vi "N9030B_8257D_0916.vi"() -> ()   [LabVIEW 2017]
uses:
  <vilib>/picture/cartesn2.llb/XY Plot Type.ctl
  <vilib>/Utility/file.llb/Write Delimited Spreadsheet (DBL).vi
  <vilib>/Utility/file.llb/Write Delimited Spreadsheet (string).vi
  <instrlib>/Keysight XSAn/Keysight XSAn.lvlib
panel:
  in  "XY Plot Cosmetics":T2(array[cluster])=[{"Color Box"=3381759, "plot type"=enum."connected squares", "baseline"=0.0}, {"Color Box"=6618880, "plot type"=enum."connected points", "baseline"=0.0}, {"Color Box"=16768018, "plot type"=enum."connected circles", "baseline"=0.0}]
  out "?":picture
  in  "csv header":string[](array[string])
  in  "folder name":string
  out "element":dbl
  out "sweep":bool
  in  "stop":bool
  in  "Path":path=path "d:/"
  out "actual points":i32
  in  "Array":cluster{"Numeric":dbl, "Numeric 2":dbl}[](array[cluster])
  in  "frequency points":T3 {"point 2 (Hz)" format="%#_6p"; "point 1 (Hz)" format="%#_6p"; "frequency 1 (Hz)" format="%#_6p"}
  in  "Keysight N9030B":refnum<visa-resource-name> caption="resource name"
  in  "8257D":refnum<visa-resource-name>
  in  "8257D":T4={"start frequency (MHz)"=150.0, "frequency spacing (MHz)"=1.0, "stop frequency (MHz)"=250.0, "sweep frequency"=FALSE, "Power level"=0.0}
  out "error out":errorcluster {"code" format="%.0x"}
  in  "Keysight N9030B":T5={"center frequency"=15000.0, "span"=5000.0, "noise floor (dBm)"=0.0} {"span" format="%#_6p"; "center frequency" format="%#_6p"}
  out "amplitude":dbl[](array[numeric])
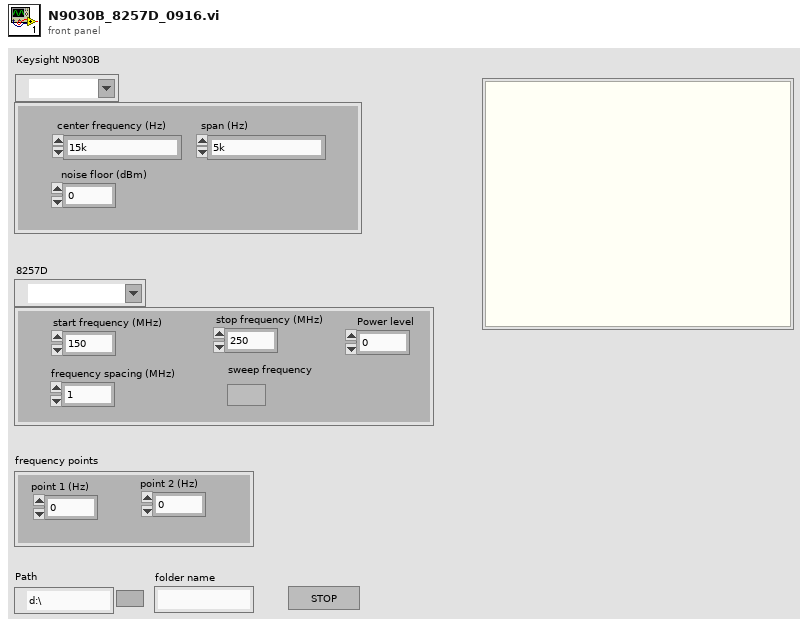
[diagram p1: front panel]
types:
  T1 = typedef "XY Plot Type.ctl" = enum16{"points", "squares", "circles", "connected points", "connected squares", "connected circles", "comb plot", "sized scatter plot", "sized-colored scatter plot", "min-max lines"}
  T2 = cluster{"Color Box":u32, "plot type":T1, "baseline":dbl}[]
  T3 = cluster{"frequency 1 (Hz)":dbl, "point 1 (Hz)":dbl, "point 2 (Hz)":dbl}
  T4 = cluster{"start frequency (MHz)":dbl, "frequency spacing (MHz)":dbl, "stop frequency (MHz)":dbl, "sweep frequency":bool, "Power level":dbl}
  T5 = cluster{"center frequency":dbl, "span":dbl, "noise floor (dBm)":dbl}
  T6 = cluster{"Array":cluster{"Numeric":dbl, "Numeric 2":dbl}[]}
  T7 = cluster{"Array":cluster{"Numeric":dbl, "Numeric 2":dbl}[]}[]
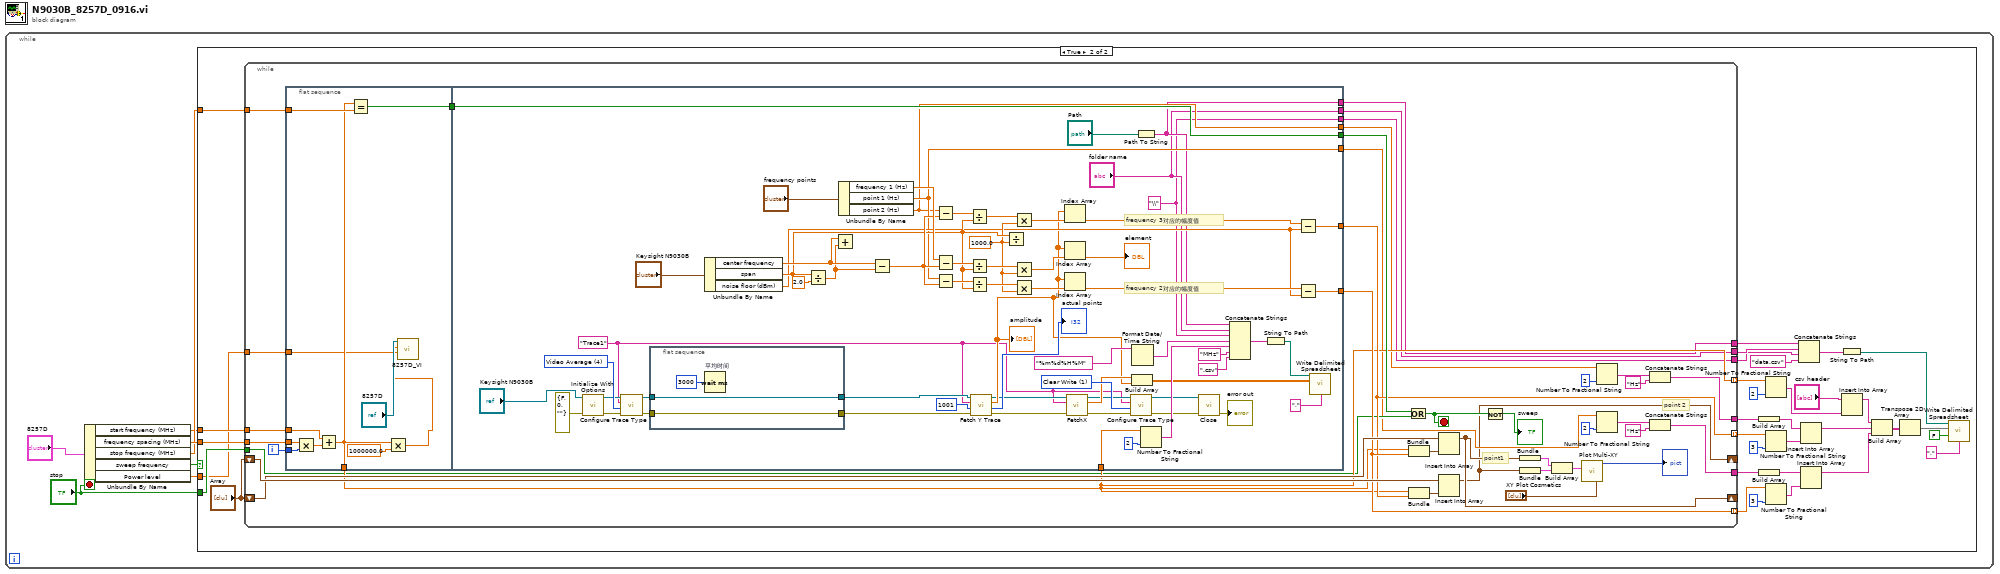
[diagram p0: block diagram]
diagram:
  n1 = while {
    stop <- "stop" stop-if-true
    n2 = Unbundle By Name("8257D") -> ("start frequency (MHz)"=w3:dbl, "frequency spacing (MHz)"=w5:dbl, "stop frequency (MHz)"=w4:dbl, "sweep frequency"=w6:bool, "Power level"=w1:dbl)
    n3 = case shown="True" w6 {
      tunnel: w3 -> [_ w38]
      tunnel: w5 -> [_ w40]
      tunnel: w4 -> [_ w37]
      tunnel: "stop" -> [_ w35]
      tunnel: w1 -> [_ w8]
      frame False {
      }
      frame True {
        n4 = while {
          tunnel: w38 -> [w77]
          tunnel: w40 -> [w76]
          tunnel: w37 -> [w74]
          shift-right: [w50] -> _
          shift-left: "Array" -> [w72]
          shift-right: [w51] -> _
          shift-left: "Array" -> [w71]
          tunnel: [w65] -> w29 mode=indexing
          tunnel: [w64] -> w18 mode=indexing
          tunnel: [w63] -> w24 mode=indexing
          tunnel: w35 -> [w62]
          tunnel: [w57] -> w31
          tunnel: [w52] -> w20
          tunnel: [w44] -> w14
          tunnel: [w43] -> w13
          tunnel: [w42] -> w12
          tunnel: w8 -> [w41]
          i -> [w75]
          stop <- w67 stop-if-true
          # "point 2"
          # "point1"
          n5 = flat-sequence {
            tunnel: w77 -> [w88]
            tunnel: w76 -> [w87]
            tunnel: w75 -> [w86]
            tunnel: w74 -> [w83]
            tunnel: [w82] -> w73
            tunnel: [w81] -> w63
            tunnel: w41 -> [w78]
            tunnel: [w152] -> w68
            tunnel: w73 -> [w152]
            tunnel: [w117] -> w65
            tunnel: [w120] -> w64
            tunnel: w63 -> [w131]
            tunnel: [w114] -> w61
            tunnel: [w113] -> w56
            tunnel: [w91] -> w44
            tunnel: ["folder name"] -> w43
            tunnel: [w89] -> w42
            frame #0 {
              n6 = Multiply(x=w87, y=w86) -> (x*y=w85:dbl)
              n7 = Add(x=w88, y=w85) -> (x+y=w81:dbl)
              n8 = Equal?(x=w81, y=w83) -> (x = y?=w82:bool)
              n9 = Multiply(x=w81, y=1000000.0) -> (x*y=w79:dbl)
              n10 = call "8257D_VI.vi"("PowerLevel"=w78, "Frequency"=w79, "8257D"="8257D") -> ()  [unwired: 3 in]
            }
            frame #1 {
              w107 = 1 items=["Clear Write"=1, "Maximum Hold"=2, "Minimum Hold"=3, "Video Average"=4, "View"=5, "Store"=6] ("trace type (Clear Write)")
              w112 = 4 items=["Clear Write"=1, "Maximum Hold"=2, "Minimum Hold"=3, "Video Average"=4, "View"=5, "Store"=6] ("trace type (Clear Write)")
              w92 = "Trace1" ("trace name")
              w89 = "\\" ("string")
              w124 = 1000.0 ("y")
              # "frequency 3对应的幅度值"
              # "frequency 2对应的幅度值"
              n11 = call <instrlib>:"Initialize With Options.vi"("error in (no error)"=errorcluster {"status"=FALSE, "code"=0, "source"=""}, "resource string"="Keysight N9030B") -> ("error out"=w110:errorcluster, "instrument handle out"=w111:refnum<k15>)  [unwired: 8 in]
              n12 = call <instrlib>:"Configure Trace Type.vi"("error in (no error)"=w110, "trace type (Clear Write)"=w112, "trace name"=w92, "instrument handle"=w111) -> ("error out"=w108:errorcluster, "instrument handle out"=w109:refnum<k15>)  [unwired: 6 in]
              n13 = flat-sequence {
                tunnel: [w153] -> w143
                tunnel: [w154] -> w144
                tunnel: w109 -> [w154]
                tunnel: w108 -> [w153]
                frame #0 {
                  n14 = Wait (ms) "平均时间"(milliseconds to wait=u32 3000) -> ()  [unwired: 1 out]
                }
              }
              n15 = Unbundle By Name("Keysight N9030B") -> ("center frequency"=w141:dbl, "span"=w126:dbl, "noise floor (dBm)"=w118:dbl)
              n16 = Divide(x=w126, y=2.0) -> (x/y=w140:dbl)
              n17 = Add(x=w141, y=w140) -> ()  [unwired: 1 out]
              n18 = Unbundle By Name("frequency points") -> ("frequency 1 (Hz)"=w129:dbl, "point 1 (Hz)"=w114:dbl, "point 2 (Hz)"=w113:dbl)
              n19 = Subtract(x=w141, y=w140) -> (x-y=w128:dbl)
              n20 = Subtract(x=w113, y=w128) -> (x-y=w136:dbl)
              n21 = Subtract(x=w129, y=w128) -> (x-y=w127:dbl)
              n22 = Subtract(x=w114, y=w128) -> (x-y=w139:dbl)
              n23 = Divide(x=w136, y=w126) -> (x/y=w135:dbl)
              n24 = Divide(x=w127, y=w126) -> (x/y=w125:dbl)
              n25 = Divide(x=w139, y=w126) -> (x/y=w138:dbl)
              n26 = call <instrlib>:"Fetch Y Trace.vi"("error in (no error)"=w143, "array length"=1001, "trace name"=w92, "instrument handle"=w144) -> ("error out"=w97:errorcluster, "actual points"=→"actual points":i32, "amplitude"=w103:dbl[], "instrument handle out"=w98:refnum<k15>)  [unwired: 4 in]
              "amplitude" <- w103
              n27 = Divide(x=w126, y=w124) -> ()  [unwired: 1 out]
              n28 = Multiply(x=w135, y=w124) -> (x*y=w134:dbl)
              n29 = Multiply(x=w125, y=w124) -> (x*y=w123:dbl)
              n30 = Multiply(x=w138, y=w124) -> (x*y=w137:dbl)
              n31 = Index Array(array=w103, index=w134) -> (element=w121:dbl)
              n32 = Index Array(array=w103, index=w123) -> (element=→"element":dbl)
              n33 = Index Array(array=w103, index=w137) -> (element=w119:dbl)
              n34 = call <instrlib>:"FetchX.vi"("error in (no error)"=w97, "Trace"=w92, "instrument handle"=w98) -> ("error out"=w95:errorcluster, "Val"=w104:dbl[], "instrument handle out"=w96:refnum<k15>)  [unwired: 5 in, 1 out]
              n35 = call <instrlib>:"Configure Trace Type.vi"("error in (no error)"=w95, "trace type (Clear Write)"=w107, "trace name"=w92, "instrument handle"=w96) -> ("error out"=w105:errorcluster, "instrument handle out"=w106:refnum<k15>)  [unwired: 6 in]
              n36 = Build Array(w104, w103) -> (w102:dbl[][])
              n37 = Format Date/Time String(time format string (%c)="%m%d%H%M") -> (date/time string=w115:string)  [unwired: 2 in]
              n38 = Path To String(path="Path") -> (string=w91:string)
              n39 = Number To Fractional String(number=w131, precision (6)=i16 2) -> (F-format string=w116:string)  [unwired: 2 in]
              n40 = call <instrlib>:"Close.vi"("error in (no error)"=w105, "instrument handle"=w106) -> ("error out"=→"error out":errorcluster)  [unwired: 9 in]
              n41 = Concatenate Strings(w91, "folder name", w89, w115, w116, "MHz" ("string"), ".csv" ("string")) -> (w100:string)
              n42 = String To Path(string=w100) -> (path=w99:path)
              n43 = Subtract(x=w121, y=w118) -> (x-y=w120:dbl)
              n44 = Subtract(x=w119, y=w118) -> (x-y=w117:dbl)
              n45 = call-poly <vilib>:"Write Delimited Spreadsheet.vi"("file path (dialog if empty)"=w99, "2D data"=w102, "delimiter (\\t)"="," ("delimiter (\\t)")) -> ()  [unwired: 11 in, 2 out]
            }
          }
          n46 = Or(x=w68, y=w62) -> (x .or. y?=w67:bool)
          n47 = Bundle(w63, w65) -> (w70:cluster{dbl, dbl})  [unwired: 1 in]
          n48 = Bundle(w63, w64) -> (w69:cluster{dbl, dbl})  [unwired: 1 in]
          n49 = Insert Into Array(array=w71, new element=w70) -> (w51:cluster{"Numeric":dbl, "Numeric 2":dbl}[])  [unwired: 1 in]
          n50 = Insert Into Array(array=w72, new element=w69) -> (w50:cluster{"Numeric":dbl, "Numeric 2":dbl}[])  [unwired: 1 in]
          n51 = Not(x=w67) -> (.not. x?=→"sweep":bool)
          n52 = Bundle("Array"=w51) -> (w49:T6)  [unwired: 1 in]
          n53 = Bundle("Array"=w50) -> (w48:T6)  [unwired: 1 in]
          n54 = Build Array(w49, w48) -> (w47:T7)
          n55 = call <vilib>:"Plot Multi-XY.vi"("data"=w47, "XY plot cosmetics"="XY Plot Cosmetics") -> ("new picture"=→"?":picture)  [unwired: 13 in]
          n56 = Number To Fractional String(number=w56, precision (6)=i16 2) -> (F-format string=w54:string)  [unwired: 2 in]
          n57 = Number To Fractional String(number=w61, precision (6)=i16 2) -> (F-format string=w59:string)  [unwired: 2 in]
          n58 = Concatenate Strings(w54, "Hz" ("string")) -> (w52:string)
          n59 = Concatenate Strings(w59, "Hz" ("string")) -> (w57:string)
        }
        n60 = Build Array(w20) -> (w19:string[])
        n61 = Build Array(w31) -> (w30:string[])
        n62 = Number To Fractional String(number=w24, precision (6)=i16 2) -> (F-format string=w22:string[])  [unwired: 2 in]
        n63 = Number To Fractional String(number=w18, precision (6)=i16 3) -> (F-format string=w16:string[])  [unwired: 2 in]
        n64 = Number To Fractional String(number=w29, precision (6)=i16 3) -> (F-format string=w27:string[])  [unwired: 2 in]
        n65 = Concatenate Strings(w14, w13, w12, "data.csv" ("string")) -> (w10:string)
        n66 = Insert Into Array(array=w19, new element=w16) -> (w15:string[])  [unwired: 1 in]
        n67 = Insert Into Array(array=w30, new element=w27) -> (w26:string[])  [unwired: 1 in]
        n68 = String To Path(string=w10) -> (path=w9:path)
        n69 = Insert Into Array(array="csv header", new element=w22) -> (w21:string[])  [unwired: 1 in]
        n70 = Build Array(w21, w15, w26) -> (w34:string[][])
        n71 = Transpose 2D Array(2D array=w34) -> (transposed array=w33:string[][])
        n72 = call-poly <vilib>:"Write Delimited Spreadsheet.vi"("file path (dialog if empty)"=w9, "2D data"=w33, "append to file? (new file:F)"=FALSE, "delimiter (\\t)"="," ("delimiter (\\t)")) -> ()  [unwired: 10 in, 2 out]
      }
    }
  }
